vi "close comm references.vi"(8 "error in (no error)":errorcluster, 9 "status queue":T1, 10 "cmd queue":T1, 11 "configuration notifier":refnum<notifier>) -> (0 "error out":errorcluster)   [LabVIEW 2014, in "Simple Sequencer TBM runtime.lvclass"]
uses:
  Simple Sequencer TBM runtime.lvclass
  configuration/Simple Sequencer TBM configuration.lvclass
  <vilib>/NI/AMC/Message Queue.ctl
  <vilib>/NI/AMC/Message.ctl
  <vilib>/NI/Tools/Keyed Array/KeyedArray.ctl
  <vilib>/NI/Tools/Keyed Array/Tools_KeyedArray.lvlib
  <vilib>/NI/AMC/AMC.lvlib
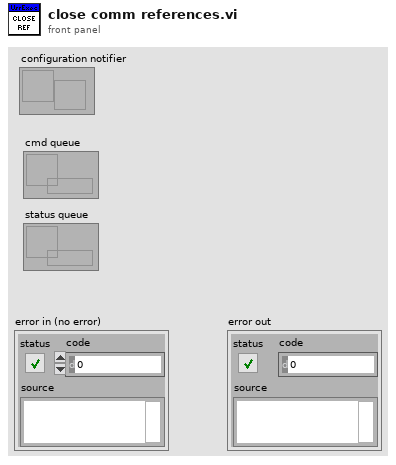
[diagram p1: front panel]
types:
  T1 = typedef "AMC.lvlib/Message Queue.ctl" = refnum<queue>
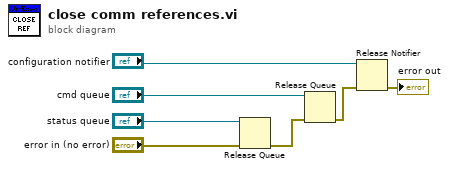
[diagram p0: block diagram]
diagram:
  n1 = Release Queue(queue="status queue", error in (no error)="error in (no error)") -> (error out=w5:errorcluster)  [unwired: 1 in, 2 out]
  n2 = Release Queue(queue="cmd queue", error in (no error)=w5) -> (error out=w6:errorcluster)  [unwired: 1 in, 2 out]
  n3 = Release Notifier(notifier="configuration notifier", error in (no error)=w6) -> (error out=→"error out":errorcluster)  [unwired: 1 in, 2 out]
